vi "bulge wall align v0.1.vi"(8 "error in (no error)":errorcluster) -> (0 "error out":errorcluster, 2 "distance":dbl)   [LabVIEW 2019]
uses:
  <vilib>/Platform/TimedLoop/XDataNode/timing_clust.ctl
  <vilib>/Platform/TimedLoop/XDataNode/nitl_modes.ctl
  <vilib>/Platform/TimedLoop/XDataNode/wakeup.ctl
  <vilib>/addons/control/pid/pid.llb/PID (DBL).vi
  <vilib>/platform/TimedLoop/XDataNode/XDataNode.xnode
  <vilib>/Platform/TimedLoop/XDataNode/XDNodeRunTimeDep.lvlib
  gyro/BNO055/class/angle Converter.lvclass
  <vilib>/addons/control/pid/NI_PID_pid.lvlib
panel:
  in  "stop":bool
  out "result":bool
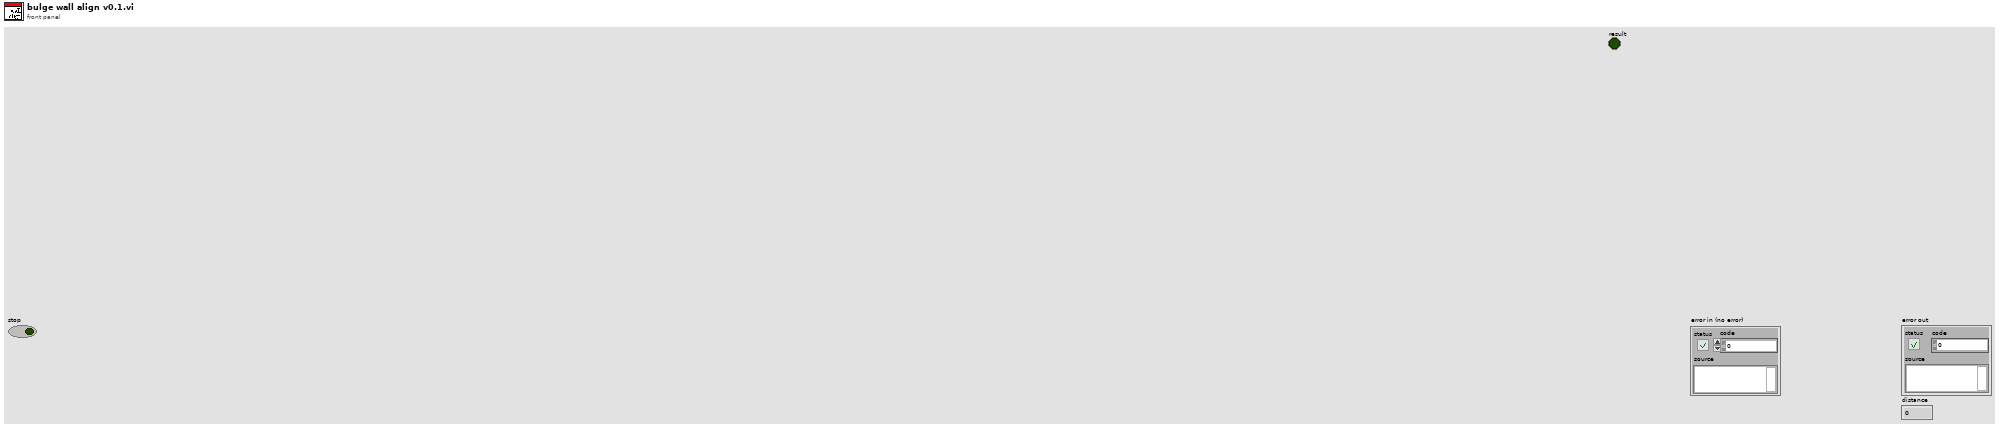
[diagram p1: front panel]
types:
  T1 = typedef "AI.lvlib/AI Reference.ctl" = cluster{"myRIO Reference":T2, "AI Channels List":T6, "AI Scaling Constants List":T8}
  T2 = typedef "myRIO Generic Hardware Reference.ctl" = cluster{"myRIO Model":T3, "myRIO Hardware Reference":T4}
  T3 = typedef "Hardware Version Enum.ctl" = enum16{"Unknown", "myRIO-1900", "myRIO-1950", "roboRIO", "NI ELVIS RIO CM", "ELVIS III"}
  T4 = typedef "myRIO v1.0 Reference.ctl" = cluster{"Generic FPGA Reference":T5, "Allow multiple opens":bool}
  T5 = typedef "Generic FPGA Reference.ctl" = refnum<k20>
  T6 = typedef "AI Channels List.ctl" = T7[]
  T7 = typedef "AI Channels Enum.ctl" = enum16{"Not Connected", "AudioIn/Left", "AudioIn/Right", "C/AI0", "C/AI1", "A/AI0", "A/AI1", "A/AI2", "A/AI3", "A/AI4", "A/AI5", "A/AI6", "A/AI7", "B/AI0", "B/AI1", "B/AI2", "B/AI3", "B/AI4", "B/AI5", "B/AI6", "B/AI7", "AI/AI0", "AI/AI1", "AI/AI2", "AI/AI3", "A/AI0 (DIFF)", "A/AI1 (DIFF)", "A/AI2 (DIFF)", "A/AI3 (DIFF)", "B/AI0 (DIFF)", "B/AI1 (DIFF)", "B/AI2 (DIFF)", "B/AI3 (DIFF)"}
  T8 = typedef "Analog Scaling Constants List.ctl" = T9[]
  T9 = typedef "Analog Scaling Constants.ctl" = cluster{"LSB Weight (Volts)":dbl, "Offset (Volts)":dbl, "Signed?":bool}
  T10 = typedef "XDNodeRunTimeDep.lvlib/timing_clust.ctl" = cluster{"Expected End [f-1]":u64, "Actual End [f-1]":u64, "Finished Late? [f-1]":bool, "Expected End [i-1]":u64, "Actual End [i-1]":u64, "Finished Late? [i-1]":bool, "Expected Start [i]":u64, "Actual Start [i]":u64, "Expected Start [f]":u64, "Actual Start [f]":u64, "Source Name":string, "Structure Name":string, "Period":i64, "Deadline":i64, "Offset":i64, "Start":i64, "Priority":i32, "Timeout":i32, "Mode":T11, "Wakeup Reason":T12, "Error":errorcluster, "Source Type":string, "Secondary Source Type":string, "Global End Time":u64, "Global Start Time":u64, "Frame Duration":u64, "Iteration Duration":u64, "Assigned CPU":i32, "I/O Scan Engine Mode":u32}
  T11 = typedef "XDNodeRunTimeDep.lvlib/nitl_modes.ctl" = enum32{"No Change", "Process missed periods, maintain original phase", "Discard missed periods, maintain original phase", "Process missed periods, ignore original phase", "Discard missed periods, ignore original phase"}
  T12 = typedef "XDNodeRunTimeDep.lvlib/wakeup.ctl" = enum32{"Normal", "Aborted", "Asynchronous wakeup", "Timing source error", "Timed loop error", "Timeout"}
  T13 = typedef "IR out.ctl" = cluster{"DC estimate (V) 2":dbl, "DC estimate (V)":dbl, "AC estimate (Vrms)":dbl, "AC estimate (Vrms) 2":dbl}
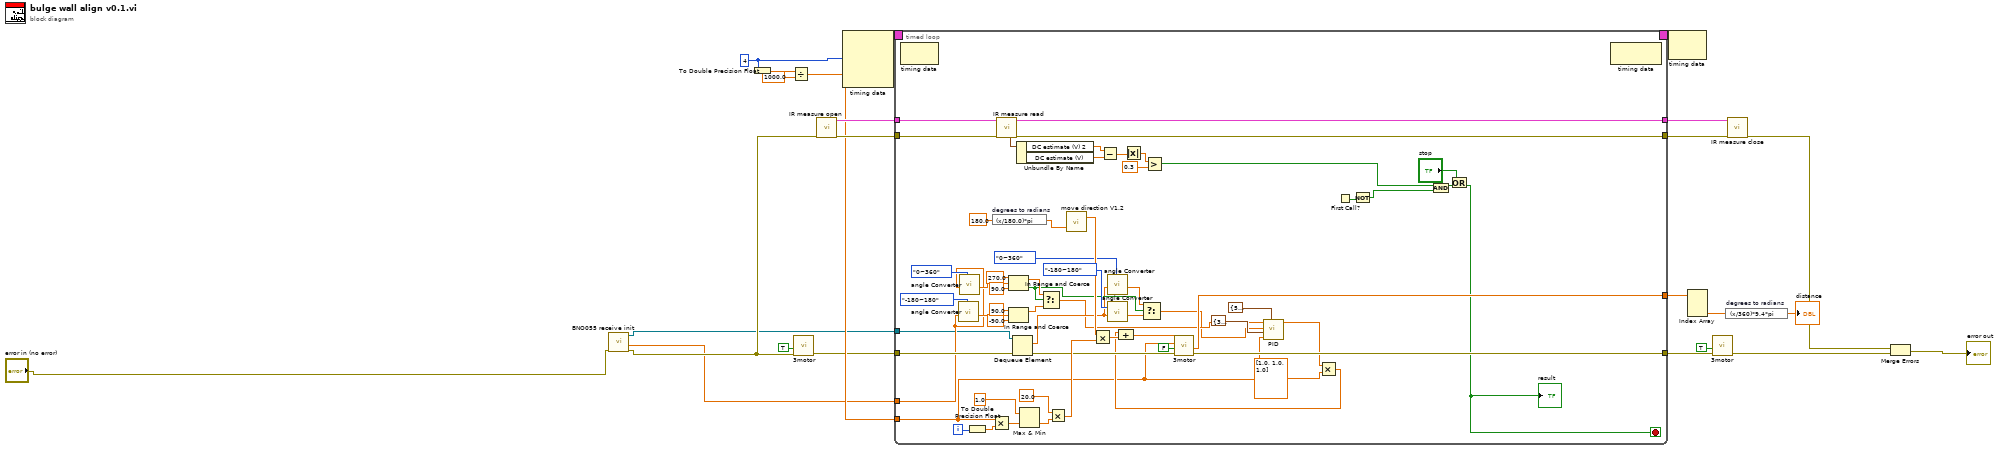
[diagram p0: block diagram]
diagram:
  w18 = i64 4 ("Period")
  n1 = call "BNO055 receive init.vi"("error in (no error)"="error in (no error)") -> ("error out"=w4:errorcluster, "element"=w1:dbl, "queue out"=w3:refnum<queue>)  [unwired: 8 in]
  n2 = To Double Precision Float(number=w18) -> (double precision float=w17:dbl)
  n3 = Divide(x=w17, y=1000.0) -> (x/y=w15:dbl)
  n4 = call "3motor.vi"("error in (no error)"=w4, "Reset"=TRUE) -> ("error out"=w13:errorcluster)  [unwired: 8 in, 1 out]
  n5 = call "IR measure open.vi"("error in (no error)"=w4) -> ("error out"=w22:errorcluster, "AI Ref Out"=w19:T1)  [unwired: 9 in]
  n6 = node-c288(w18) -> (w24:T10)  [unwired: 3 in]
  n7 = timed-loop {
    timing: w24 -> [_]
    timing-out: [_] -> w23
    tunnel: w22 -> [w83]
    tunnel: [w82] -> w21
    tunnel: [w81] -> w20
    tunnel: w19 -> [w80]
    tunnel: w15 -> [w26]
    tunnel: [w71] -> w14
    tunnel: w13 -> [w39]
    tunnel: [w57] -> w7
    tunnel: w1 -> [w37]
    tunnel: w3 -> [w36]
    i -> [w77]
    stop <- w29 stop-if-true
    n8 = node-c288() -> ()  [unwired: 1 in, 1 out]
    n9 = call "angle Converter.vi"("select"=enum16{"-180~180", "0~360"}."-180~180", "input angle"=w37) -> ("angle out"=w47:dbl)  [unwired: 9 in]
    n10 = call "angle Converter.vi"("select"=enum16{"-180~180", "0~360"}."0~360", "input angle"=w37) -> ("angle out"=w50:dbl)  [unwired: 9 in]
    n11 = To Double Precision Float(number=w77) -> (double precision float=w76:dbl)
    n12 = Multiply(x=w26, y=w76) -> (x*y=w75:dbl)
    n13 = expression code="(x/180.0)*pi" "degrees to radians"(180.0) -> (w79:dbl)
    n14 = call "IR measure read.vi"("error in (no error)"=w83, "AI Ref In"=w80) -> ("error out"=w82:errorcluster, "AI Ref Out"=w81:T1, "output cluster"=w64:T13)  [unwired: 6 in, 1 out]
    n15 = In Range and Coerce(upper limit=270.0, x=w50, lower limit=90.0) -> (coerced(x)=w46:dbl, In Range?=w41:bool)
    n16 = In Range and Coerce(upper limit=90.0, x=w47, lower limit=-90.0) -> (coerced(x)=w45:dbl)  [unwired: 1 out]
    n17 = Dequeue Element(queue=w36, error in (no error)=w39) -> (element=w40:dbl, error out=w38:errorcluster)  [unwired: 1 in, 2 out]
    n18 = Unbundle By Name(w64) -> ("DC estimate (V) 2"=w62:dbl, "DC estimate (V)"=w63:dbl)
    n19 = Max & Min(x=1.0, y=w75) -> (min(x,y)=w73:dbl)  [unwired: 1 out]
    n20 = Select(t=w46, s=w41, f=w45) -> (s? t:f=w33:dbl)
    n21 = Multiply(x=20.0, y=w73) -> (x*y=w68:dbl)
    n22 = call "move direction V1.2.vi"("theta"=w79) -> ("out array"=w69:dbl[])  [unwired: 1 in, 1 out]
    n23 = Multiply(x=w69, y=w68) -> (x*y=w70:dbl[])
    n24 = Subtract(x=w62, y=w63) -> (x-y=w61:dbl)
    n25 = call "angle Converter.vi"("select"=enum16{"-180~180", "0~360"}."-180~180", "input angle"=w40) -> ("angle out"=w42:dbl)  [unwired: 9 in]
    n26 = call "angle Converter.vi"("select"=enum16{"-180~180", "0~360"}."0~360", "input angle"=w40) -> ("angle out"=w43:dbl)  [unwired: 9 in]
    n27 = Absolute Value(x=w61) -> (abs(x)=w60:dbl)
    n28 = Select(t=w43, s=w41, f=w42) -> (s? t:f=w27:dbl)
    n29 = Greater?(x=w60, y=0.3) -> (0:w58:bool)
    n30 = call-poly <vilib>:"PID.vi"("output range"=cluster{"output high":dbl, "output low":dbl} {"output high"=50.0, "output low"=-50.0}, "dt (s)"=w26, "PID gains"=cluster{"Kp":dbl, "Ki":dbl, "Kd":dbl} {"Kp"=3.0, "Ki"=0.0, "Kd"=0.002} ("PID"), "process variable"=w27, "setpoint"=w33) -> ("output"=w25:dbl)  [unwired: 5 in, 1 out]
    n31 = Multiply(x=w25, y=dbl[] [1.0, 1.0, 1.0]) -> (x*y=w31:dbl[])
    n32 = Compound Arithmetic op=ADD(w31, w70) -> (w56:dbl[])
    n33 = call "3motor.vi"("error in (no error)"=w38, "Reset"=FALSE, "dt(s)"=w26, "Motor speed"=w56) -> ("error out"=w71:errorcluster, "process"=w57:dbl[])  [unwired: 6 in]
    n34 = First Call?() -> (First Call?: T/F=w66:bool)
    n35 = Not(x=w66) -> (.not. x?=w65:bool)
    n36 = And(x=w58, y=w65) -> (x .and. y?=w55:bool)
    n37 = Or(x="stop", y=w55) -> (x .or. y?=w29:bool)
    "result" <- w29
    n38 = node-c288() -> ()  [unwired: 1 in, 1 out]
  }
  n39 = node-c288(w23) -> ()  [unwired: 1 out]
  n40 = Index Array(array=w7) -> (element #3=w6:dbl)  [unwired: 3 in, 2 out]
  n41 = call "3motor.vi"("error in (no error)"=w14, "Reset"=TRUE) -> ("error out"=w10:errorcluster)  [unwired: 8 in, 1 out]
  n42 = expression code="(x/360)*9.4*pi" "degrees to radians"(w6) -> (→"distance":dbl)
  n43 = call "IR measure close.vi"("error in (no error)"=w21, "AI Ref In"=w20) -> ("error out"=w8:errorcluster)  [unwired: 9 in]
  n44 = Merge Errors(w8, w10) -> (→"error out":errorcluster)
